vi "Generate_WayPoints_Hopping_CV_Surface_and_Bulk.vi"(11 "Input Cluster":T2={"Scan Rate (um/s)"=15.0, "X Start"=15.0, "X End"=15.0, "Y Start"=15.0, "Y End"=15.0, " Z Start"=15.0, "HoppingDistance"=1.0, "V"=15.0, "Z End"=15.0, "Approach Rate Hopping (um/s)"=15.0, "Retrack Rate (um/s)"=15.0, "V 2"=15.0, "Approach Rate (um/s)"=15.0, "CV Rate / V/s"=15.0, "V 1"=15.0, "HoldTime1/s"=15.0, "Hold time 2 / s"=15.0}) -> (0 "output cluster":T1)   [LabVIEW 2023]
uses:
  TypeDefs/WayPointCluster.ctl
  User_Vi/Settings.vi
panel:
  in  "WayPointCluster":T1
  out "Y  P":dbl
  out "X  P":dbl
  out "HoppingDistanceX":dbl
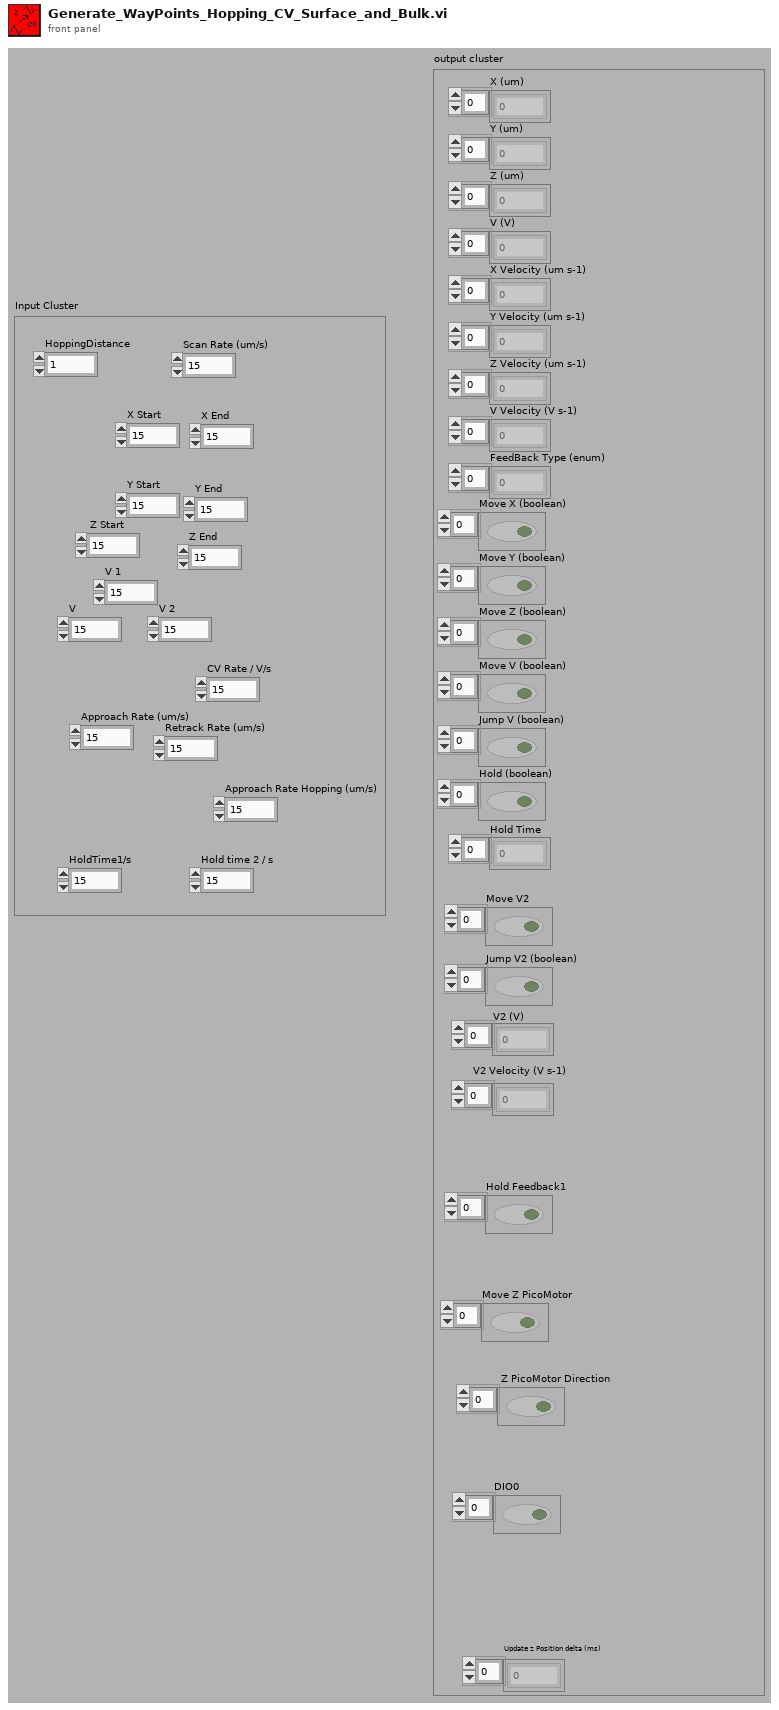
[diagram p1: front panel]
types:
  T1 = typedef "WayPointCluster.ctl" = cluster{"X (um)":dbl[], "Y (um)":dbl[], "Z (um)":dbl[], "V (V)":dbl[], "X Velocity (um s-1)":dbl[], "Y Velocity (um s-1)":dbl[], "Z Velocity (um s-1)":dbl[], "V Velocity (V s-1)":dbl[], "FeedBack Type (enum)":u16[], "Move X (boolean)":bool[], "Move Y (boolean)":bool[], "Move Z (boolean)":bool[], "Move V (boolean)":bool[], "Jump V (boolean)":bool[], "Hold (boolean)":bool[], "Hold Time":u32[], "V2 (V)":dbl[], "Move V2":bool[], "V2 Velocity (V s-1)":dbl[], "Jump V2 (boolean)":bool[], "Update z Position delta (ms)":i16[], "Hold Feedback1":bool[], "Move Z PicoMotor":bool[], " Z PicoMotor Direction":bool[], "DIO0":bool[]}
  T2 = cluster{"Scan Rate (um/s)":dbl, "X Start":dbl, "X End":dbl, "Y Start":dbl, "Y End":dbl, " Z Start":dbl, "HoppingDistance":dbl, "V":dbl, "Z End":dbl, "Approach Rate Hopping (um/s)":dbl, "Retrack Rate (um/s)":dbl, "V 2":dbl, "Approach Rate (um/s)":dbl, "CV Rate / V/s":dbl, "V 1":dbl, "HoldTime1/s":dbl, "Hold time 2 / s":dbl}
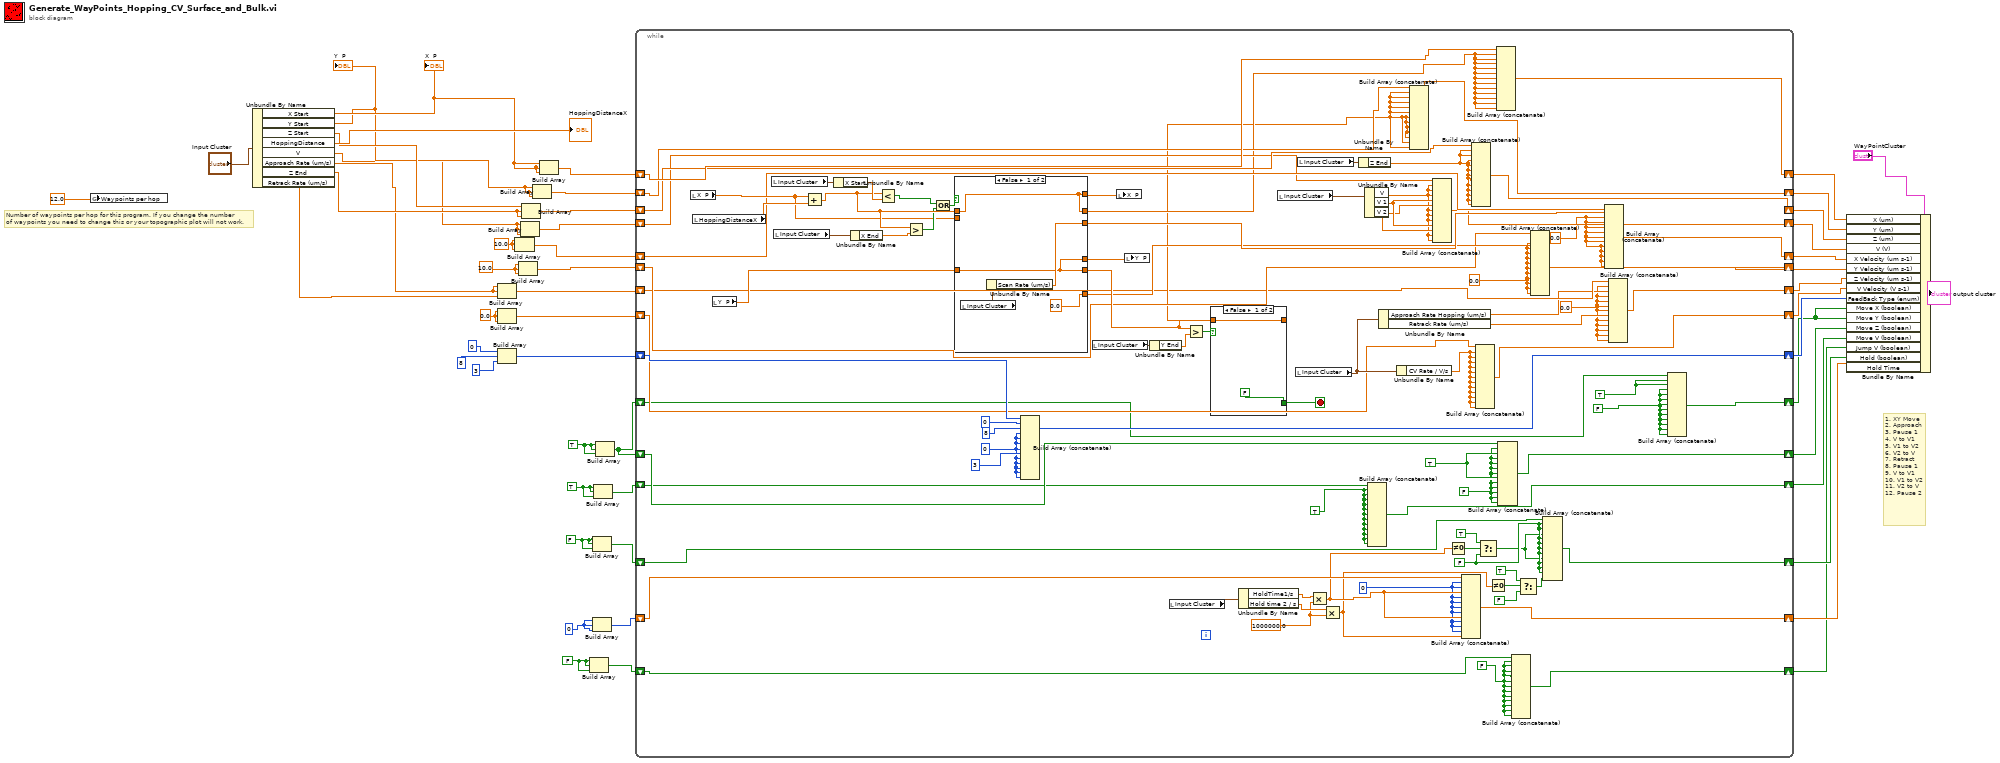
[diagram p0: block diagram]
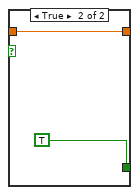
[diagram p2: hidden frame]
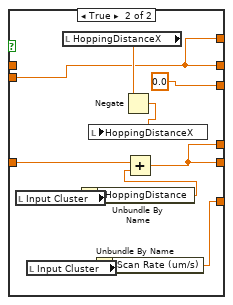
[diagram p3: hidden frame]
diagram:
  w14 = FALSE
  w18 = FALSE
  w17 = u32 0 ("element")
  w16 = TRUE
  w12 = TRUE
  w8 = 10.0 ("element")
  w9 = 10.0 ("element")
  w11 = 0.0 ("element")
  # "Number of waypoints per hop for this program. If you change the number\nof waypoints you need to change this or your topographic plot will not work."
  # "1. XY Move\n2. Approach\n3. Pause 1\n4. V to V1\n5. V1 to V2\n6. V2 to V\n7. Retract\n8. Pause 1\n9. V to V1\n10. V1 to V2\n11. V2 to V\n12. Pause 2"
  n1 = global write "Settings.vi" "Waypoints per hop"(12.0) -> ()
  n2 = Unbundle By Name("Input Cluster") -> ("X Start"=w31:dbl, "Y Start"=w30:dbl, "Z Start"=w32:dbl, "HoppingDistance"=→"HoppingDistanceX":dbl, "V"=w28:dbl, "Approach Rate (um/s)"=w10:dbl, "Z End"=w29:dbl, "Retrack Rate (um/s)"=w27:dbl)
  "X  P" <- w31
  "Y  P" <- w30
  n3 = Build Array(w10, w10, w27) -> (w39:dbl[])
  n4 = Build Array(u16 0 ("element"), u16 8 ("element"), u16 3 ("element")) -> (w35:u16[])
  n5 = Build Array(w11, w11, w11) -> (w37:dbl[])
  n6 = Build Array(w8, w8, w8) -> (w42:dbl[])
  n7 = Build Array(w9, w9, w9) -> (w41:dbl[])
  n8 = Build Array(w28, w28, w28) -> (w44:dbl[])
  n9 = Build Array(w32, w29, w29) -> (w46:dbl[])
  n10 = Build Array(w30, w30, w30) -> (w48:dbl[])
  n11 = Build Array(w31, w31, w31) -> (w50:dbl[])
  n12 = Build Array(w18, w18, w18) -> (w21:bool[])
  n13 = Build Array(w14, w14, w14) -> (w13:bool[])
  n14 = Build Array(w17, w17, w17) -> (w24:u32[])
  n15 = Build Array(w16, w16, w16) -> (w20:bool[])
  n16 = Build Array(w12, w12, w12) -> (w4:bool[])
  n17 = while {
    shift-right: [w118] -> w49
    shift-left: w50 -> [w119]
    shift-right: [w116] -> w47
    shift-left: w48 -> [w117]
    shift-right: [w114] -> w45
    shift-left: w46 -> [w115]
    shift-right: [w107] -> w43
    shift-left: w44 -> [w108]
    shift-right: [w106] -> w25
    shift-left: w42 -> [w113]
    shift-right: [w109] -> w40
    shift-left: w41 -> [w110]
    shift-right: [w105] -> w38
    shift-left: w39 -> [w76]
    shift-right: [w103] -> w36
    shift-left: w37 -> [w104]
    shift-right: [w138] -> w34
    shift-left: w35 -> [w139]
    shift-right: [w101] -> w23
    shift-left: w4 -> [w102]
    shift-right: [w97] -> w3
    shift-left: w13 -> [w98]
    shift-right: [w95] -> w22
    shift-left: w24 -> [w96]
    shift-right: [w90] -> w2
    shift-left: w21 -> [w91]
    shift-right: [w99] -> w15
    shift-left: w20 -> [w100]
    shift-right: [w87] -> w5
    shift-left: w4 -> [w86]
    stop <- w126 stop-if-true
    w71 = FALSE
    w88 = TRUE
    w89 = 1000000.0 ("y")
    w77 = 0.0 ("element")
    w68 = TRUE
    w56 = FALSE
    w57 = u32 0 ("element")
    w65 = FALSE
    w69 = FALSE
    w70 = TRUE
    w83 = u16 0 ("element")
    w55 = 0.0 ("element")
    w73 = 0.0 ("element")
    n18 = local read "X  P"() -> (w125:dbl)
    n19 = local read "HoppingDistanceX"() -> (w140:dbl)
    n20 = local read "Y  P"() -> (w124:dbl)
    n21 = local read "Input Cluster"() -> (w142:T2)
    n22 = local read "Input Cluster"() -> (w141:T2)
    n23 = Add(x=w125, y=w140) -> (x+y=w132:dbl)
    n24 = Unbundle By Name(w142) -> ("X Start"=w135:dbl)
    n25 = Unbundle By Name(w141) -> ("X End"=w133:dbl)
    n26 = Less?(x=w132, y=w135) -> (x < y?=w134:bool)
    n27 = Greater?(x=w132, y=w133) -> (0:w131:bool)
    n28 = Or(x=w134, y=w131) -> (x .or. y?=w130:bool)
    n29 = case shown="False" w130 {
      tunnel: w132 -> [w147 _]
      tunnel: [w147 w153] -> w82
      tunnel: w125 -> [_ w153]
      tunnel: w124 -> [w148 w154]
      tunnel: [w148 w152] -> w123
      tunnel: [w150 0.0] -> w112
      tunnel: [0.0 w155] -> w111
      tunnel: [w148 w152] -> w122
      tunnel: [w147 w153] -> w121
      frame False {
        n30 = local read "Input Cluster"() -> (w151:T2)
        n31 = Unbundle By Name(w151) -> ("Scan Rate (um/s)"=w150:dbl)
      }
      frame True {
        n32 = local read "Input Cluster"() -> (w159:T2)
        n33 = local read "Input Cluster"() -> (w157:T2)
        n34 = local read "HoppingDistanceX"() -> (w161:dbl)
        n35 = Unbundle By Name(w159) -> ("HoppingDistance"=w158:dbl)
        n36 = Unbundle By Name(w157) -> ("Scan Rate (um/s)"=w155:dbl)
        n37 = Negate(x=w161) -> (-x=w160:dbl)
        n38 = local write "HoppingDistanceX"(w160) -> ()
        n39 = Add(x=w154, y=w158) -> (x+y=w152:dbl)
      }
    }
    n40 = Build Array (concatenate)(w139, u16 0 ("element"), u16 8 ("element"), w83, w83, w83, w83, u16 3 ("element"), w83, w83, w83, w83, w83) -> (w138:u16[])
    n41 = local read "Input Cluster"() -> (w129:T2)
    n42 = local write "X  P"(w121) -> ()
    n43 = local write "Y  P"(w122) -> ()
    n44 = Unbundle By Name(w129) -> ("Y End"=w128:dbl)
    n45 = local read "Input Cluster"() -> (w94:T2)
    n46 = Greater?(x=w123, y=w128) -> (0:w127:bool)
    n47 = case shown="False" w127 {
      tunnel: w123 -> [w144 w146]
      tunnel: [w144 w146] -> w81
      tunnel: [FALSE TRUE] -> w126
      frame False {
      }
      frame True {
      }
    }
    n48 = Unbundle By Name(w94) -> ("HoldTime1/s"=w93:dbl, "Hold time 2 / s"=w92:dbl)
    n49 = local read "Input Cluster"() -> (w136:T2)
    n50 = local read "Input Cluster"() -> (w120:T2)
    n51 = local read "Input Cluster"() -> (w137:T2)
    n52 = Multiply(x=w93, y=w89) -> (x*y=w59:dbl)
    n53 = Multiply(x=w92, y=w89) -> (x*y=w58:dbl)
    n54 = Unbundle By Name(w137) -> ("Z End"=w80:dbl)
    n55 = Unbundle By Name(w136) -> ("V"=w54:dbl, "V 1"=w79:dbl, "V 2"=w78:dbl)
    n56 = Build Array (concatenate)(w100, w68, w68, w68, w68, w68, w68, w68, w68, w68, w68, w68, w68) -> (w99:bool[])
    n57 = Unbundle By Name(w120) -> ("Approach Rate Hopping (um/s)"=w75:dbl, "Retrack Rate (um/s)"=w74:dbl)
    n58 = Unbundle By Name(w120) -> ("CV Rate / V/s"=w72:dbl)
    n59 = Build Array (concatenate)(w117, w81, w81, w81, w81, w81, w81, w81, w81, w81, w81, w81, w81) -> (w116:dbl[])
    n60 = Build Array (concatenate)(w108, w54, w54, w54, w79, w78, w54, w54, w54, w79, w78, w54, w54) -> (w107:dbl[])
    n61 = Not Equal To 0?(x=w59) -> (x != 0?=w67:bool)
    n62 = Build Array (concatenate)(w96, w57, w57, w59, w57, w57, w57, w57, w59, w57, w57, w57, w58) -> (w95:dbl[])
    n63 = Build Array (concatenate)(w115, w80, w80, w80, w80, w80, w80, w80, w80, w80, w80, w80, w80) -> (w114:dbl[])
    n64 = Build Array (concatenate)(w104, w72, w72, w72, w72, w72, w72, w72, w72, w72, w72, w72, w72) -> (w103:dbl[])
    n65 = Select(t=TRUE, s=w67, f=w65) -> (s? t:f=w64:bool)
    n66 = Not Equal To 0?(x=w58) -> (x != 0?=w63:bool)
    n67 = Build Array (concatenate)(w119, w82, w82, w82, w82, w82, w82, w82, w82, w82, w82, w82, w82) -> (w118:dbl[])
    n68 = Build Array (concatenate)(w102, w69, w70, w69, w69, w69, w69, w70, w69, w69, w69, w69, w69) -> (w101:bool[])
    n69 = Build Array (concatenate)(w91, w56, w56, w56, w56, w56, w56, w56, w56, w56, w56, w56, w56) -> (w90:bool[])
    n70 = Select(t=TRUE, s=w63, f=FALSE) -> (s? t:f=w60:bool)
    n71 = Build Array (concatenate)(w110, w111, w55, w55, w55, w55, w55, w55, w55, w55, w55, w55, w55) -> (w109:dbl[])
    n72 = Build Array (concatenate)(w98, w65, w65, w64, w65, w65, w65, w65, w64, w65, w65, w65, w60) -> (w97:bool[])
    n73 = Build Array (concatenate)(w113, w112, w77, w77, w77, w77, w77, w77, w77, w77, w77, w77, w77) -> (w106:dbl[])
    n74 = Build Array (concatenate)(w76, w73, w75, w73, w73, w73, w73, w74, w73, w73, w73, w73, w73) -> (w105:dbl[])
    n75 = Build Array (concatenate)(w86, w88, w88, w71, w71, w71, w71, w71, w71, w71, w71, w71, w71) -> (w87:bool[])
  }
  n76 = Bundle By Name(cluster="WayPointCluster", "X (um)"=w49, "Y (um)"=w47, "Z (um)"=w45, "V (V)"=w43, "X Velocity (um s-1)"=w25, "Y Velocity (um s-1)"=w40, "Z Velocity (um s-1)"=w38, "V Velocity (V s-1)"=w36, "FeedBack Type (enum)"=w34, "Move X (boolean)"=w5, "Move Y (boolean)"=w5, "Move Z (boolean)"=w23, "Move V (boolean)"=w15, "Jump V (boolean)"=w2, "Hold (boolean)"=w3, "Hold Time"=w22) -> (→"output cluster":T1)
